vi "Read Props.vi"(8 "error in (no error)":errorcluster, 11 "BooleanIndicatorEditorPanel in":refnum<class "BooleanIndicatorEditorPanel.lvclass">) -> (0 "error out":errorcluster, 2 "Props":T1, 3 "BooleanIndicatorEditorPanel out":refnum<class "BooleanIndicatorEditorPanel.lvclass">)   [LabVIEW 2020, in "VolatusGUIControls.lvlib" / "BooleanIndicatorEditorPanel.lvclass"]
uses:
  BooleanIndicatorEditorPanel.lvclass
  BooleanIndicatorEditorPanel.lvclass/BooleanIndicatorEditorPanel.ctl
  JSON Props.ctl
  VolatusGUIEditorCore/Label Props.ctl
  VolatusGUIEditorCore/VolatusGUIEditorCore.lvlib
  VolatusGUIEditorCore/Position Props.ctl
  VolatusGUIEditorCore/Boolean Color Props.ctl
  VolatusGUIEditorCore/Boolean Text Props.ctl
  Props.ctl
  VolatusGUIControls.lvlib
  a192962a-188f-4a11-8137-c06f55f15e8d.vi
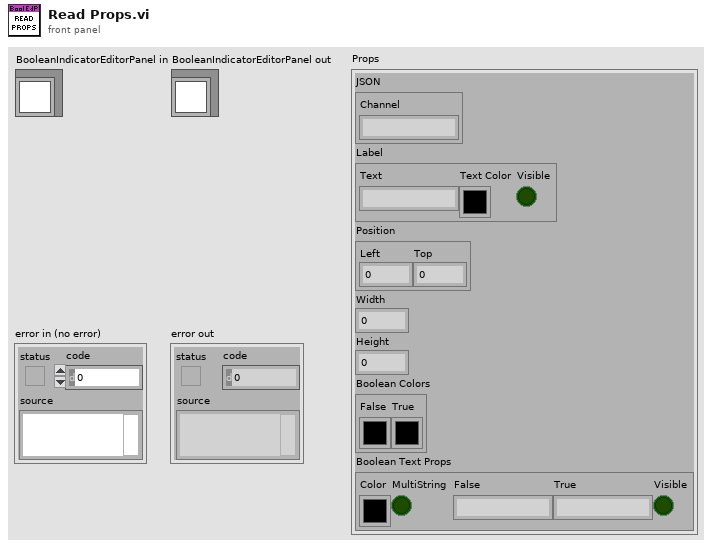
[diagram p1: front panel]
types:
  T1 = typedef "VolatusGUIControls.lvlib/BooleanIndicatorEditorPanel.lvclass/Props.ctl" = cluster{"JSON":T2, "Label":T3, "Position":T4, "Width":u16, "Height":u16, "Boolean Colors":T5, "Boolean Text Props":T6}
  T2 = typedef "VolatusGUIControls.lvlib/BooleanIndicatorEditorPanel.lvclass/JSON Props.ctl" = cluster{"Channel":string}
  T3 = typedef "VolatusGUIEditorCore.lvlib/Label Props.ctl" = cluster{"Text":string, "Text Color":u32, "Visible":bool}
  T4 = typedef "VolatusGUIEditorCore.lvlib/Position Props.ctl" = cluster{"Left":i32, "Top":i32}
  T5 = typedef "VolatusGUIEditorCore.lvlib/Boolean Color Props.ctl" = cluster{"False":u32, "True":u32}
  T6 = typedef "VolatusGUIEditorCore.lvlib/Boolean Text Props.ctl" = cluster{"Color":u32, "MultiString":bool, "False":string, "True":string, "Visible":bool}
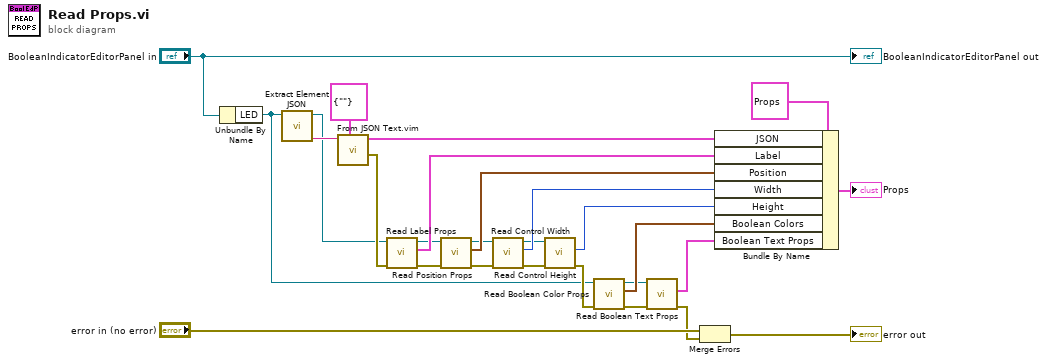
[diagram p0: block diagram]
diagram:
  n1 = Unbundle By Name("BooleanIndicatorEditorPanel in") -> ("LED"=w7:refnum<vi>)
  n2 = call "Extract Element JSON.vi"("Ctl Refnum in"=w7) -> ("JSON"=w21:string, "Ctl Refnum"=w18:refnum<vi>)  [unwired: 7 in, 2 out]
  n3 = call "From JSON Text.vim"("Data Type and Default Value"=T2 {"Channel"=""} ("JSON Props"), "JSON"=w21) -> ("error out"=w26:errorcluster, "Data out"=w19:T2)  [unwired: 8 in]
  n4 = call "Read Label Props.vi"("error in (no error)"=w26, "Ctl Refnum in"=w18) -> ("error out"=w16:errorcluster, "Label Props"=w17:T3, "Ctl Refnum"=w15:refnum<vi>)  [unwired: 7 in]
  n5 = call "Read Position Props.vi"("error in (no error)"=w16, "Ctl Refnum in"=w15) -> ("error out"=w13:errorcluster, "Position Props"=w14:T4, "Ctl Refnum"=w12:refnum<vi>)  [unwired: 7 in]
  n6 = call "Read Control Width.vi"("error in"=w13, "Control in"=w12) -> ("error out"=w10:errorcluster, "Width"=w11:u32, "Control"=w9:refnum<vi>)  [unwired: 7 in]
  n7 = call "Read Control Height.vi"("error in"=w10, "Control in"=w9) -> ("error out"=w27:errorcluster, "Height"=w8:u32)  [unwired: 7 in, 1 out]
  n8 = call "Read Boolean Color Props.vi"("error in (no error)"=w27, "Control in"=w7) -> ("error out"=w4:errorcluster, "Boolean Colors Props"=w6:T5, "Control"=w5:refnum<vi>)  [unwired: 7 in]
  n9 = call "Read Boolean Text Props.vi"("error in (no error)"=w4, "Control In"=w5) -> ("error out"=w1:errorcluster, "Boolean Text Props"=w3:T6)  [unwired: 7 in, 1 out]
  n10 = Merge Errors("error in (no error)", w1) -> (→"error out":errorcluster)
  n11 = Bundle By Name(cluster=T1 {"JSON"={"Channel"=""}, "Label"={"Text"="", "Text Color"=0, "Visible"=FALSE}, "Position"={"Left"=0, "Top"=0}, "Width"=0, "Height"=0, "Boolean Colors"={"False"=0, "True"=0}, "Boolean Text Props"={"Color"=0, "MultiString"=FALSE, "False"="", "True"="", "Visible"=FALSE}} ("Props"), "JSON"=w19, "Label"=w17, "Position"=w14, "Width"=w11, "Height"=w8, "Boolean Colors"=w6, "Boolean Text Props"=w3) -> (→"Props":T1)
  "BooleanIndicatorEditorPanel out" <- "BooleanIndicatorEditorPanel in"
